vi "Launcher.vi"   [LabVIEW 2023]
uses:
  SpectroscopyUI.lvclass
  Applications/National Instruments/LabVIEW 2023 64-bit/vi.lib/ActorFramework/Actor/Actor.lvclass
  <vilib>/ActorFramework/Actor/Actor.lvclass
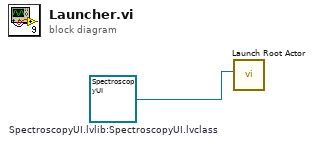
[diagram p0: block diagram]
diagram:
  w1 = refnum<class "SpectroscopyUI.lvclass"> refnum  # SpectroscopyUI.lvlib:SpectroscopyUI.lvclass
  n1 = call <vilib>:"Launch Root Actor.vi"("Actor"=w1) -> ()  [unwired: 9 in, 2 out]
